vi "laucher.vi"() -> ()   [LabVIEW 2011]
panel:
  out "Loading":u8(slide) scale=0.0..100.0
  # "HPTS Of  VNA Automatic Measurement System"
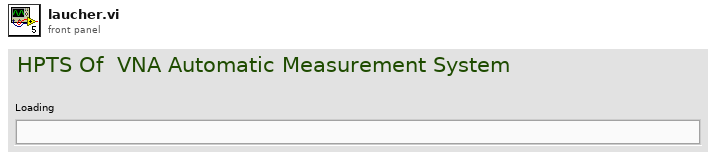
[diagram p1: front panel]
types:
  T1 = enum32{"Invalid", "Standard", "Closed", "Hidden", "Minimized", "Maximized"}
  T2 = enum16{"Always On", "Always Off", "Off While Running"}
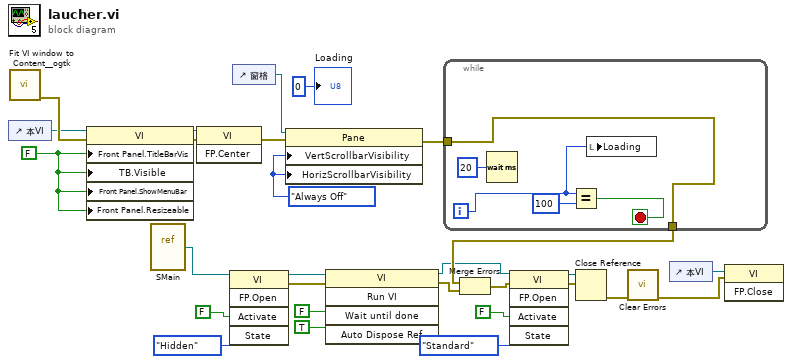
[diagram p0: block diagram]
diagram:
  w27 = T2."Always Off" ("垂直滚动条可见")
  w25 = FALSE ("前面板窗口:标题栏可见")
  n1 = control-ref of="本VI"() -> (w24:refnum<vi>)
  n2 = call <userlib>:"Fit VI window to Content__ogtk.vi"() -> ("error out"=w28:errorcluster)  [unwired: 6 in, 1 out]
  n3 = property class="VI"(reference=w24, error in=w28, "Front Panel.TitleBarVis"=w25, "TB.Visible"=w25, "Front Panel.ShowMenuBar"=w25, "Front Panel.Resizeable"=w25) -> (reference out=w23:refnum<vi>, error out=w22:errorcluster)
  n4 = vi-ref "SMain.vi"() -> (w1:refnum<vi>)
  n5 = invoke class="VI" method="FP.Center"(reference=w23, error in=w22) -> (error out=w21:errorcluster)  [unwired: 1 in, 2 out]
  n6 = invoke class="VI" method="FP.Open"(reference=w1, "Activate"=FALSE ("激活？"), "State"=T1."Hidden" ("状态")) -> (reference out=w19:refnum<vi>, error out=w12:errorcluster)  [unwired: 2 in, 3 out]
  n7 = control-ref of="窗格"() -> (w3:refnum<vi>)
  n8 = property class="Pane"(reference=w3, error in=w21, "VertScrollbarVisibility"=w27, "HorizScrollbarVisibility"=w27) -> (error out=w26:errorcluster)  [unwired: 1 out]
  n9 = invoke class="VI" method="Run VI"(reference=w19, error in=w12, "Wait until done"=FALSE ("结束前等待"), "Auto Dispose Ref"=TRUE ("自动销毁引用")) -> (reference out=w7:refnum<vi>, error out=w10:errorcluster)  [unwired: 1 in, 3 out]
  n10 = while {
    tunnel: w26 -> [w30]
    tunnel: [w30] -> w11
    i -> [w29]
    stop <- w31 stop-if-true
    n11 = Wait (ms)(milliseconds to wait=u32 20 ("等待时间（毫秒）")) -> ()  [unwired: 1 out]
    n12 = Equal?(x=w29, y=100) -> (x = y?=w31:bool)
    n13 = local write "Loading"(w29) -> ()
  }
  n14 = Merge Errors(w11, w10) -> (w6:errorcluster)
  n15 = invoke class="VI" method="FP.Open"(reference=w7, error in=w6, "Activate"=FALSE ("激活？"), "State"=T1."Standard" ("状态")) -> (reference out=w9:refnum<vi>, error out=w8:errorcluster)  [unwired: 1 in, 3 out]
  n16 = Close Reference(reference=w9, error in (no error)=w8) -> (error out=w16:errorcluster)
  n17 = call <vilib>:"Clear Errors.vi"("error in (no error)"=w16) -> ("error out"=w15:errorcluster)  [unwired: 6 in]
  n18 = control-ref of="本VI"() -> (w17:refnum<vi>)
  n19 = invoke class="VI" method="FP.Close"(reference=w17, error in=w15) -> ()  [unwired: 1 in, 3 out]
  "Loading" <- u8 0 ("水平进度条")
